vi "Local Configuration.DMAMODE0.Done Interrupt Enable.Get.vi"(8 "error in (no error)":errorcluster, 11 "GE 5565PIORC":refnum<class "GE 5565PIORC.lvclass">) -> (0 "error out":errorcluster, 2 "Done Interrupt Enabled?":bool, 3 "GE 5565PIORC out":refnum<class "GE 5565PIORC.lvclass">)   [LabVIEW 2016, in "GE 5565PIORC.lvclass"]
uses:
  GE 5565PIORC.lvclass
  GE 5565PIORC.lvclass/GE 5565PIORC.ctl
  <vilib>/Instr/_visa.llb/VISA Register Access Address Space.ctl
  Controls/Registers.Local Configuration.ctl
  Binary Operations/Get Bits U32.vi
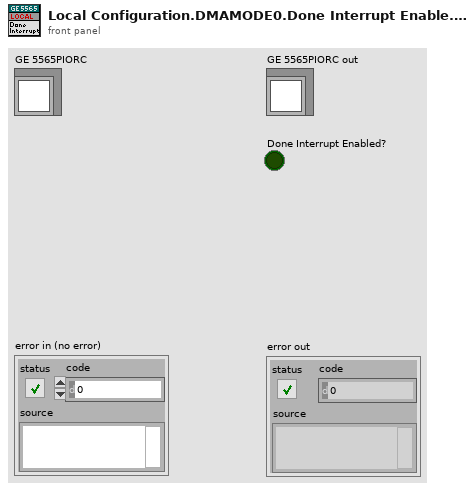
[diagram p1: front panel]
types:
  T1 = typedef "GE 5565PIORC.lvclass/Registers.Local Configuration.ctl" = u32
  T2 = typedef "VISA Register Access Address Space.ctl" = u16
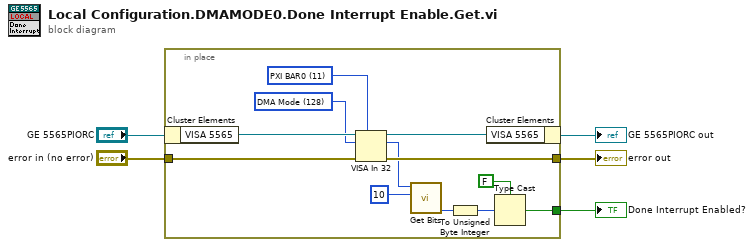
[diagram p0: block diagram]
diagram:
  n1 = in-place {
    in-place-border: "error in (no error)" -> [w15]
    in-place-border: [w14] -> w3
    in-place-border: [w6] -> w1
    w10 = T1 128 items=["INTCSR"=104, "DMA Mode"=128, "DMA PCI Address"=132, "DMA Local Address"=136, "DMA Transfer Byte Count"=140, "DMA Descriptor Pointer"=144, "DMA CSR 0"=168, "DMA PCI DAC Upper Address"=180, "PCI PIO Address Range"=240, "PCI PIO Base Address (Remap)"=244] ("Local Configration Register Offset")
    w11 = T2 11 items=["VXI/VME A16"=1, "VXI/VME A24"=2, "VXI/VME A32"=3, "VXI/VME A64"=4, "PXI Memory Allocations"=9, "PXI Configuration"=10, "PXI BAR0"=11, "PXI BAR1"=12, "PXI BAR2"=13, "PXI BAR3"=14, "PXI BAR4"=15, "PXI BAR5"=16] ("Address Space")
    n2 = in-place-cluster #1("GE 5565PIORC") -> ("VISA 5565"=w17:refnum<visa-resource-name>)
    n3 = VISA In 32(7:w11, 8:w15, 10:w10, 11:w17) -> (0:w14:errorcluster, 2:w13:u32, 3:w16:refnum<visa-resource-name>)
    n4 = call-poly "Get Bits.vi"("Start Index (0)"=u8 10, "Register in"=w13) -> ("Value"=w9:u32)  [unwired: 6 in, 3 out]
    n5 = To Unsigned Byte Integer(number=w9) -> (unsigned 8bit integer=w8:u8)
    n6 = in-place-cluster #1("VISA 5565"=w16) -> (→"GE 5565PIORC out":refnum<class "GE 5565PIORC.lvclass">)
    n7 = Type Cast(type=FALSE, x=w8) -> (*(type *) &x=w6:bool)
  }
  "error out" <- w3
  "Done Interrupt Enabled?" <- w1
